vi "Function.vi"(8 "error in (no error)":errorcluster, 10 "A":T1, 11 "NOT_I64.lvclass":refnum<class "NOT_I64.lvclass">) -> (0 "error out":errorcluster, 2 "Result":T1, 3 "NOT out":refnum<class "NOT_I64.lvclass">)   [LabVIEW 2021, in "NOT_I64.lvclass"]
uses:
  NOT_I64.lvclass
  Type.ctl
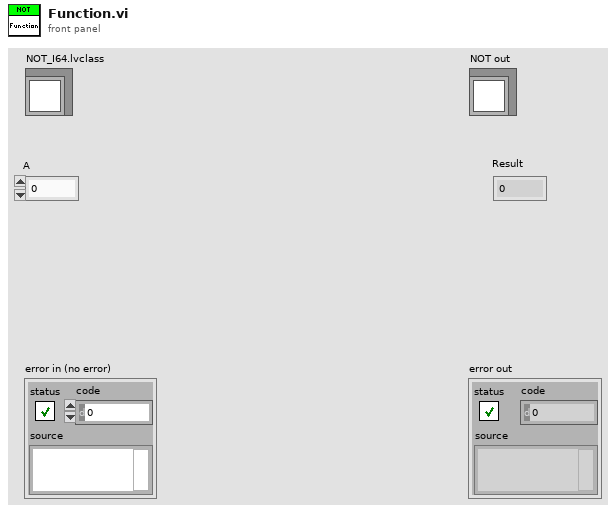
[diagram p1: front panel]
types:
  T1 = typedef "NOT_I64.lvclass/Type.ctl" = i64
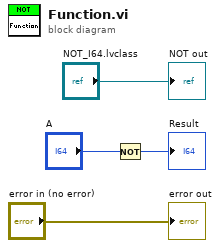
[diagram p0: block diagram]
diagram:
  n1 = Not(x="A") -> (.not. x?=→"Result":T1)
  "error out" <- "error in (no error)"
  "NOT out" <- "NOT_I64.lvclass"
